vi "Set Shared Memory Size.vi"(8 "error in (no error)":errorcluster, 10 "size (bytes)":u32, 11 "shared memory in":T1) -> (0 "error out":errorcluster, 3 "shared memory out":T1)   [LabVIEW 2013, in "Linux RT IPC.lvlib" / "Shared Memory.lvlib" / "Shared Memory.lvclass"]
doc: "This VI allows the size of the shared memory file to be set to a certain number of bytes. Memory operations are more efficient when the allocated memory is some multiple of the system page size. Use this VI in conjunction with the Get System Page Size VI to set the size of the shared memory to be a multiple of the page size."
uses:
  Shared Memory.lvclass
  Controls/reference.ctl
  Shared Memory.lvclass/Shared Memory.ctl
  Controls/file mode.ctl
  C/C.lvlib
  Shared Memory.lvlib
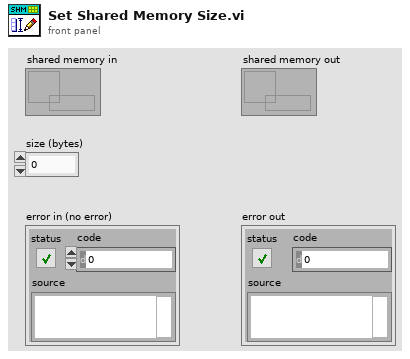
[diagram p1: front panel]
types:
  T1 = typedef "Linux RT IPC.lvlib/Shared Memory.lvlib/reference.ctl" = refnum<data-value>
  T2 = typedef "Linux RT IPC.lvlib/Shared Memory.lvlib/file mode.ctl" = enum16{"open", "create/replace"}
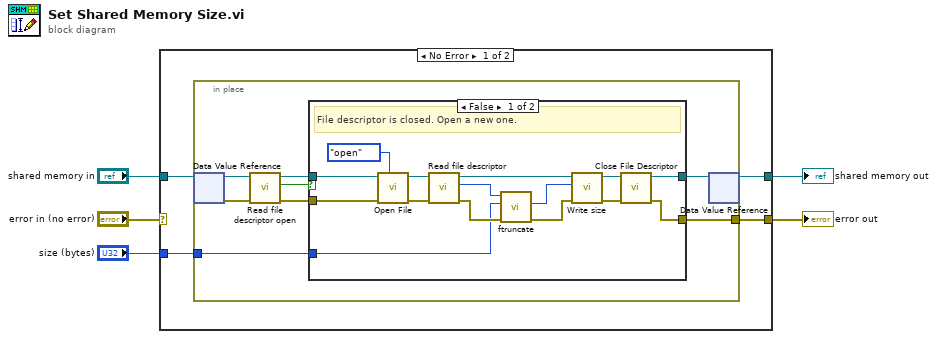
[diagram p0: block diagram]
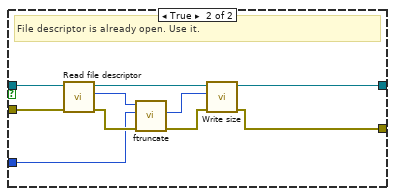
[diagram p2: hidden frame]
diagram:
  n1 = case shown="No Error" "error in (no error)" {
    selector: "error in (no error)" -> [_ w43]
    tunnel: "shared memory in" -> [w9 w44]
    tunnel: [w8 w43] -> w2
    tunnel: [w7 w44] -> w4
    tunnel: "size (bytes)" -> [w6 _]
    frame No Error {
      n2 = in-place {
        in-place-border: [w16] -> w8
        in-place-border: w6 -> [w15]
        n3 = in-place-dvr #1(w9) -> (w14:refnum<class "Shared Memory.lvclass">, w13:errorcluster)
        n4 = call "Read file descriptor open.vi"("error in (no error)"=w13, "Shared Memory in"=w14) -> ("error out"=w11:errorcluster, "file descriptor open"=w10:bool, "Shared Memory out"=w12:refnum<class "Shared Memory.lvclass">)  [unwired: 7 in]
        n5 = case shown="False" w10 {
          tunnel: w12 -> [w30 w37]
          tunnel: [w32 w36] -> w17
          tunnel: w11 -> [w29 w35]
          tunnel: [w31 w34] -> w16
          tunnel: w15 -> [w18 w33]
          frame False {
            # "File descriptor is closed. Open a new one."
            n6 = call "Open File.vi"("file mode"=file_mode."open", "error in (no error)"=w29, "Shared Memory in"=w30) -> ("error out"=w21:errorcluster, "Shared Memory out"=w22:refnum<class "Shared Memory.lvclass">)  [unwired: 7 in]
            n7 = call "Read file descriptor.vi"("error in (no error)"=w21, "Shared Memory in"=w22) -> ("error out"=w25:errorcluster, "file descriptor"=w24:i32, "Shared Memory out"=w23:refnum<class "Shared Memory.lvclass">)  [unwired: 7 in]
            n8 = call "ftruncate.vi"("error in (no error)"=w25, "size (bytes)"=w18, "file descriptor"=w24) -> ("error out"=w27:errorcluster, "size (bytes)"=w26:u32)  [unwired: 6 in, 1 out]
            n9 = call "Write size.vi"("error in (no error)"=w27, "size (bytes)"=w26, "Shared Memory in"=w23) -> ("error out"=w19:errorcluster, "Shared Memory out"=w20:refnum<class "Shared Memory.lvclass">)  [unwired: 7 in]
            n10 = call "Close File Descriptor.vi"("error in (no error)"=w19, "Shared Memory in"=w20) -> ("error out"=w31:errorcluster, "Shared Memory out"=w32:refnum<class "Shared Memory.lvclass">)  [unwired: 8 in]
          }
          frame True {
            # "File descriptor is already open. Use it."
            n11 = call "Read file descriptor.vi"("error in (no error)"=w35, "Shared Memory in"=w37) -> ("error out"=w40:errorcluster, "file descriptor"=w39:i32, "Shared Memory out"=w38:refnum<class "Shared Memory.lvclass">)  [unwired: 7 in]
            n12 = call "ftruncate.vi"("error in (no error)"=w40, "size (bytes)"=w33, "file descriptor"=w39) -> ("error out"=w42:errorcluster, "size (bytes)"=w41:u32)  [unwired: 6 in, 1 out]
            n13 = call "Write size.vi"("error in (no error)"=w42, "size (bytes)"=w41, "Shared Memory in"=w38) -> ("error out"=w34:errorcluster, "Shared Memory out"=w36:refnum<class "Shared Memory.lvclass">)  [unwired: 7 in]
          }
        }
        n14 = in-place-dvr #1(w17) -> (w7:T1)  [unwired: 1 out]
      }
    }
    frame Error {
    }
  }
  "error out" <- w2
  "shared memory out" <- w4
